vi "Update.vi"(8 "error in (no error)":errorcluster, 10 "Message in":refnum<class "UpdateMessage.lvclass">, 11 "ImageStack in":refnum<class "ImageStack.lvclass">) -> (0 "error out":errorcluster, 3 "ImageStack out":refnum<class "ImageStack.lvclass">)   [LabVIEW 2012, in "ImageStack.lvclass"]
doc: "The update method processes the command 'update'. \n\nThe command 'update' is used for receiving new values to be set to the private data of the class. This could be seen as a public set method for setting new parameters to the private class data."
uses:
  ImageStack.lvclass
  <vilib>/Distrio/Murmex/UpdateMessage/UpdateMessage.lvclass
  ImageStack.lvclass/ImageStack.ctl
  <vilib>/Distrio/Murmex/Murmex/Murmex.lvclass
panel:
  # "This method is called when the UPDATE\ntrigger is sent. \n\nOverride this method when your component needs to\nrespond to this trigger. \n\nCall parent for proper implementation"
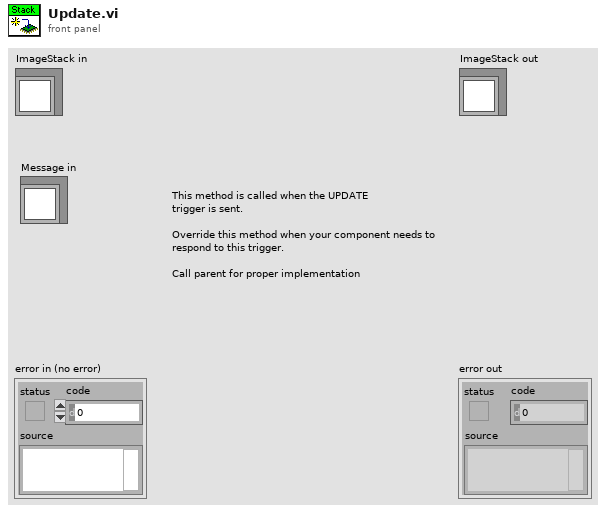
[diagram p1: front panel]
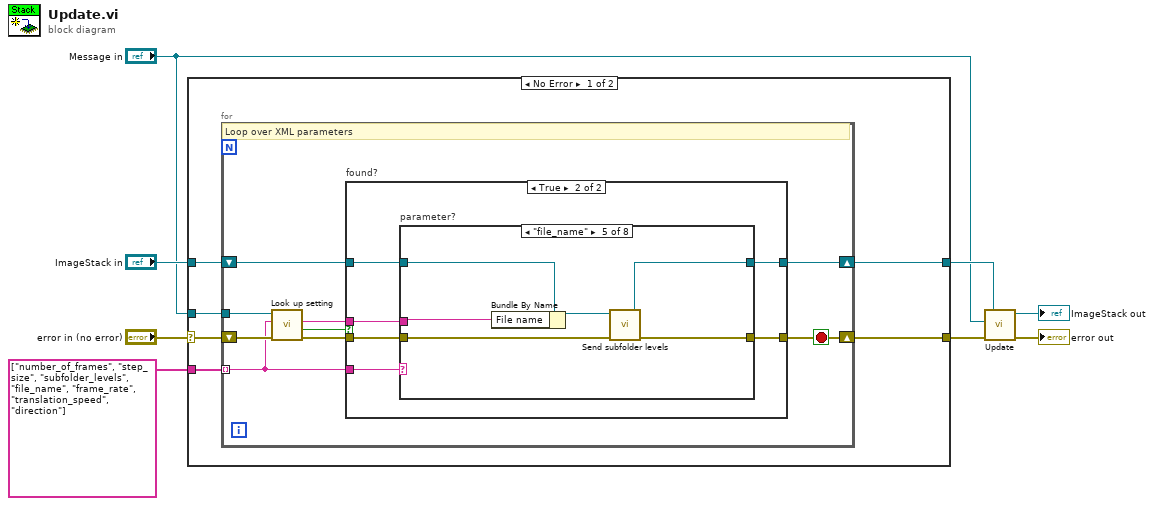
[diagram p0: block diagram]
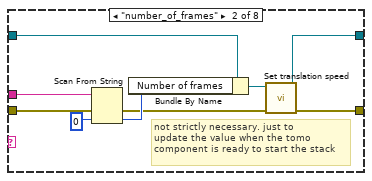
[diagram p4: hidden frame]
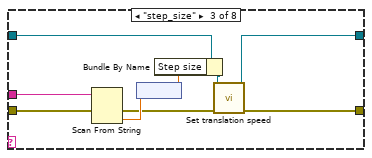
[diagram p5: hidden frame]
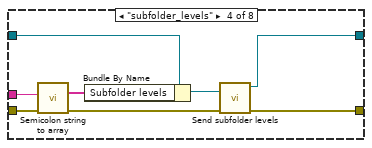
[diagram p6: hidden frame]
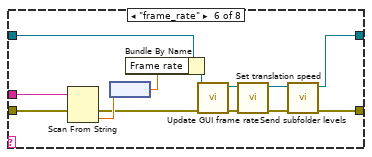
[diagram p7: hidden frame]
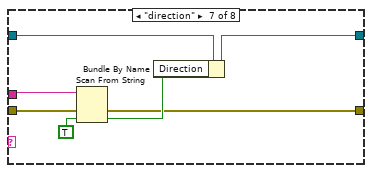
[diagram p8: hidden frame]
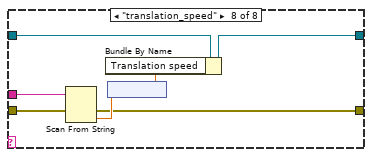
[diagram p9: hidden frame]
diagram:
  n1 = case shown="No Error" "error in (no error)" {
    selector: "error in (no error)" -> [w14 w94]
    tunnel: [w9 w94] -> w1
    tunnel: [w12 w93] -> w6
    tunnel: "ImageStack in" -> [w13 w93]
    tunnel: "Message in" -> [w11 _]
    tunnel: string[] ["number_of_frames", "step_size", "subfolder_levels", "file_name", "frame_rate", "translation_speed", "direction"] -> [w10 _]
    frame No Error {
      n2 = for {
        shift-right: [w15] -> w9
        shift-left: w14 -> [w22]
        shift-right: [w16] -> w12
        shift-left: w13 -> [w18]
        tunnel: w11 -> [w23]
        tunnel: w10 -> [w17] mode=indexing
        stop <- w15 stop-if-true
        # "Loop over XML parameters"
        n3 = call <vilib>:"Look up setting.vi"("error in (no error)"=w22, "tag name"=w17, "UpdateMessage in"=w23) -> ("error out"=w20:errorcluster, "found?"=w21:bool, "value"=w19:string)  [unwired: 5 in, 1 out]
        n4 = case "found?" shown="True" w21 {
          tunnel: w20 -> [w24 w29]
          tunnel: w19 -> [_ w30]
          tunnel: w18 -> [w25 w28]
          tunnel: w17 -> [_ w31]
          tunnel: [w24 w27] -> w15
          tunnel: [w25 w26] -> w16
          frame False {
          }
          frame True {
            n5 = case "parameter?" shown="\"file_name\"" w31 {
              tunnel: w30 -> [_ w42 w51 w58 w64 w74 w83 w87]
              tunnel: w29 -> [w32 w41 w50 w57 w63 w78 w85 w90]
              tunnel: w28 -> [w33 w39 w49 w59 w65 w75 w82 w88]
              tunnel: [w32 w36 w44 w54 w62 w67 w80 w89] -> w27
              tunnel: [w33 w34 w43 w53 w60 w68 w79 w86] -> w26
              frame Default {
              }
              frame "number_of_frames" {
                # "not strictly necessary. just to\nupdate the value when the tomo\ncomponent is ready to start the stack"
                n6 = Scan From String(input string=w42, error in=w41, default 1=u16 0) -> (error out=w37:errorcluster, output 1=w38:u16)  [unwired: 2 in, 2 out]
                n7 = Bundle By Name(cluster=w39, "Number of frames"=w38) -> (w35:refnum<class "ImageStack.lvclass">)
                n8 = call-dynamic "Set translation speed.vi"("error in (no error)"=w37, "ImageStack in"=w35) -> ("error out"=w36:errorcluster, "ImageStack out"=w34:refnum<class "ImageStack.lvclass">)  [unwired: 8 in]
              }
              frame "step_size" {
                n9 = Scan From String(input string=w51, error in=w50) -> (error out=w45:errorcluster, output 1=w48:dbl)  [unwired: 3 in, 2 out]
                n10 = node(w48) -> (w47:dbl[unit])
                n11 = Bundle By Name(cluster=w49, "Step size"=w47) -> (w46:refnum<class "ImageStack.lvclass">)
                n12 = call-dynamic "Set translation speed.vi"("error in (no error)"=w45, "ImageStack in"=w46) -> ("error out"=w44:errorcluster, "ImageStack out"=w43:refnum<class "ImageStack.lvclass">)  [unwired: 8 in]
              }
              frame "subfolder_levels" {
                n13 = call "Semicolon string to array.vi"("error in"=w57, "Semicolon string"=w58) -> ("error out"=w55:errorcluster, "String array"=w56:string[])  [unwired: 8 in]
                n14 = Bundle By Name(cluster=w59, "Subfolder levels"=w56) -> (w52:refnum<class "ImageStack.lvclass">)
                n15 = call-dynamic "Send subfolder levels.vi"("error in (no error)"=w55, "ImageStack in"=w52) -> ("error out"=w54:errorcluster, "ImageStack out"=w53:refnum<class "ImageStack.lvclass">)  [unwired: 8 in]
              }
              frame "file_name" {
                n16 = Bundle By Name(cluster=w65, "File name"=w64) -> (w61:refnum<class "ImageStack.lvclass">)
                n17 = call-dynamic "Send subfolder levels.vi"("error in (no error)"=w63, "ImageStack in"=w61) -> ("error out"=w62:errorcluster, "ImageStack out"=w60:refnum<class "ImageStack.lvclass">)  [unwired: 8 in]
              }
              frame "frame_rate" {
                n18 = Scan From String(input string=w74, error in=w78) -> (error out=w73:errorcluster, output 1=w76:dbl)  [unwired: 3 in, 2 out]
                n19 = node(w76) -> (w77:dbl[unit])
                n20 = Bundle By Name(cluster=w75, "Frame rate"=w77) -> (w71:refnum<class "ImageStack.lvclass">)
                n21 = call-dynamic "Update GUI frame rate.vi"("error in (no error)"=w73, "ImageStack in"=w71) -> ("error out"=w72:errorcluster, "ImageStack out"=w70:refnum<class "ImageStack.lvclass">)  [unwired: 8 in]
                n22 = call-dynamic "Set translation speed.vi"("error in (no error)"=w72, "ImageStack in"=w70) -> ("error out"=w66:errorcluster, "ImageStack out"=w69:refnum<class "ImageStack.lvclass">)  [unwired: 8 in]
                n23 = call-dynamic "Send subfolder levels.vi"("error in (no error)"=w66, "ImageStack in"=w69) -> ("error out"=w67:errorcluster, "ImageStack out"=w68:refnum<class "ImageStack.lvclass">)  [unwired: 8 in]
              }
              frame "direction" {
                n24 = Scan From String(input string=w83, error in=w85, default 1=TRUE) -> (error out=w80:errorcluster, output 1=w81:bool)  [unwired: 2 in, 2 out]
                n25 = Bundle By Name(cluster=w82, "Direction"=w81) -> (w79:refnum<class "ImageStack.lvclass">)
              }
              frame "translation_speed" {
                n26 = Scan From String(input string=w87, error in=w90) -> (error out=w89:errorcluster, output 1=w91:dbl)  [unwired: 3 in, 2 out]
                n27 = node(w91) -> (w92:dbl[unit])
                n28 = Bundle By Name(cluster=w88, "Translation speed"=w92) -> (w86:refnum<class "ImageStack.lvclass">)
              }
            }
          }
        }
      }
    }
    frame Error {
    }
  }
  n29 = call-parent "Update.vi"("error in (no error)"=w1, "Message in"="Message in", "Murmex in"=w6) -> ("error out"=→"error out":errorcluster, "Murmex out"=→"ImageStack out":refnum<class "ImageStack.lvclass">)  [unwired: 7 in]
